vi "ReadStrains_v200128_A.vi"() -> ()   [LabVIEW 2017]
doc: "I. Description:\nThis example demonstrates how to make continuous, hardware-timed temperature measurement using a thermocouple.\n\nII. Instructions for Running:\n1. Specify the Physical Channel where you have connected the thermocouple.\n2. Enter the Minimum and Maximum temperature values in degrees C you expect to measure. A smaller range will allow a more accurate measurement.\n3. Enter the scan rate at which you want to run the acquisition.\n4. Specify the type of thermocouple you are using.\n5. Thermocouple measurements require cold-junction compensation (CJC) to correctly scale them. Specify the source of your cold-junction compensation.\n6. If your CJC source is \"Internal\", skip the rest of the steps.\n7. If your CJC source is \"Constant Value\", specify the value (usually room temperature) in degrees C.\n8. If your CJC source is \"Channel\", specify the CJC Channel name. \n9. Specify the appropriate Auto Zero Mode. See your device's hardware manual to find out if your device supports this attribute.\n\nIII. Block Diagram Steps:\n1. Create a Thermocouple (TC) temperature measurement channel.\n2. Get all the channels in the task.\n3. Convert channel(s) array to a comma-delimited channel string.\n4. This attribute is set to compensate for input offset errors. May not be supported by all devices*.\n5. Call the Timing VI to specify the hardware timing parameters. Use device's internal clock, continuous mode acquisition and the sample rate specified by the user.\n6. Call the Start VI to program and start the acquisition.\n7. Read N samples and plot it. By default, the Read VI reads all available samples, but you can specify how many samples to read at a time and the timeout value. Continue reading data until the stop button is pressed or an error occurs. \n8. Call the Clear Task VI to clear the Task.\n9. Use the popup dialog box to display an error if any.\n\n* If your device does not support Auto Zero Mode bypass Step 2, 3, and 4.\n\nIV. I/O Connections Overview:\nConnect your thermocouple to the terminals corresponding to the Physical Channel I/O Control value."
uses:
  <vilib>/Utility/error.llb/DialogType.ctl
  <vilib>/DAQmx/read.llb/DAQmx Read (Analog 1D Wfm NChan NSamp).vi
  <vilib>/Analysis/baseanly.llb/Mean (DBL).vi
  <vilib>/Waveform/WDTOps.llb/WDT Index Channel DBL.vi
  <vilib>/DAQmx/create/channels.llb/DAQmx Create Channel (AI-Voltage-Basic).vi
  <vilib>/DAQmx/configure/timing.llb/DAQmx Timing (Sample Clock).vi
  <vilib>/DAQmx/miscellaneous.llb/DAQmx Fill In Error Info.vi
  <vilib>/Analysis/NI_AALBase.lvlib
  <vilib>/ptbypt/NI_PtbyPt.lvlib
  <vilib>/Utility/miscctls.llb/LVRowAndColumnTypeDef.ctl
panel:
  in  "Data Tag":dbl=99.0 format="%.2p"
  out "Load Cell Min Peak":dbl format="%0.2f"
  out "Load Cell Max Peak":dbl format="%0.2f"
  in  "Stop":bool
  in  "Color Box":u32(colorbox)=16448250
  out "Results":i32[](listbox)
  in  "num_chans":i32=4
  in  "Search Strings":string[](array[string])=["Verbose Name", "Units", "Sensitivity", "Offset"]
  out "TRQ_2SPD_OT (N·m)":dbl=-0.01305389404296875 format="%0.3f"
  out "Power_OT (W)":dbl=-4.779110606064606 format="%.2f"
  out "rpm_out/rpm_in":dbl=-8.382425226893735e-05 format="%.3g"
  out "AI Consumer Iterations":i32=46
  in  "path":path=path "D:/LabView Data"
  out "P2 - P1":dbl=2.2560862731933593 format="%.3f"
  out "Recorded Blocks":dbl=46.0
  in  "Force Record":bool caption="Force Record Enable"
  out "data 2":waveform(dbl)[](array[waveform])=[{"t0"=timestamp(3650018127.9917235 s since 1904-01-01), "dt"=0.1, "Y"=[0.021594634133905076, 0.022275858634939055], "attributes"=variant("NI_ChannelName"=variant(string "Dev1/ai0"), "NI_UnitDescription"=variant(string "Volts"))}, {"t0"=timestamp(3650018127.9917235 s since 1904-01-01), "dt"=0.1, "Y"=[2.0002340930725198, 1.9998772609501023], "attributes"=variant("NI_ChannelName"=variant(string "Dev1/ai0"), "NI_UnitDescription"=variant(string "Volts"))}, {"t0"=timestamp(3650018127.9917235 s since 1904-01-01), "dt"=0.1, "Y"=[1.9878001157523826, 1.9871643057998443], "attributes"=variant("NI_ChannelName"=variant(string "Dev1/ai0"), "NI_UnitDescription"=variant(string "Volts"))}, {"t0"=timestamp(3650018127.9917235 s since 1904-01-01), "dt"=0.1, "Y"=[0.006912624203864532, 0.006889916720453561], "attributes"=variant("NI_ChannelName"=variant(string "Dev1/ai0"), "NI_UnitDescription"=variant(string "Volts"))}, {"t0"=timestamp(3650018127.9917235 s since 1904-01-01), "dt"=0.1, "Y"=[0.0, 0.0], "attributes"=variant("NI_ChannelName"=variant(string "Dev1/ai0"), "NI_UnitDescription"=variant(string "Volts"))}]
  out "Power_IN (W)":dbl=0.0005711775684961294 format="%.2g"
  out "TRQ_2SPD_DRVLN_OT (N·m)":dbl=-0.018612060546874976 format="%0.3f"
  out "Waveform Chart":waveform(dbl)[](graph)=[{"t0"=timestamp(3663084502.027375 s since 1904-01-01), "dt"=0.1, "Y"=[-0.17066702696318498, -0.13693019437081472], "attributes"=variant("NI_ChannelName"=variant(string "HS_2210_STRAIN_A_POUNDS"), "NI_UnitDescription"=variant(string "lbf"))}, {"t0"=timestamp(3663084502.027375 s since 1904-01-01), "dt"=0.1, "Y"=[-50.01120067249004, -50.01071408355846], "attributes"=variant("NI_ChannelName"=variant(string "T1_OIL_OT"), "NI_UnitDescription"=variant(string "°C"))}, {"t0"=timestamp(3663084502.027375 s since 1904-01-01), "dt"=0.1, "Y"=[-0.013838771793185324, -0.013803088604682188], "attributes"=variant("NI_ChannelName"=variant(string "HS_2210_STRAIN_B_VOLTS"), "NI_UnitDescription"=variant(string "V"))}, {"t0"=timestamp(3663084502.027375 s since 1904-01-01), "dt"=0.1, "Y"=[10.033860995992347, 10.033912900500356], "attributes"=variant("NI_ChannelName"=variant(string "HS_2210_EXC_B_VOLTS"), "NI_UnitDescription"=variant(string "V"))}, {"t0"=timestamp(3663084502.027375 s since 1904-01-01), "dt"=0.1, "Y"=[1.48, 1.48], "attributes"=variant("NI_ChannelName"=variant(string "RPM_RATIO"), "NI_UnitDescription"=variant(string "ratio"))}, {"t0"=timestamp(3663084502.027375 s since 1904-01-01), "dt"=0.1, "Y"=[99.0, 99.0], "attributes"=variant("NI_ChannelName"=variant(string "DataTag"), "NI_UnitDescription"=variant(string "none"))}, {"t0"=timestamp(3663084502.027375 s since 1904-01-01), "dt"=0.1, "Y"=[0.0, 0.0], "attributes"=variant("NI_ChannelName"=variant(string "LV_CMD_2SPD_OIL_SLND"), "NI_UnitDescription"=variant(string "boolean"))}]
  in  "Run Letter":string="a"
  out "Recording":bool
  in  "Num_Blocks":dbl=100.0
  in  "Maximum Value":dbl=10.0 format="%0.2f"
  in  "Minimum Value":dbl=-10.0 format="%0.2f"
  in  "Physical Channel":tag="Dev1/ai0:3" caption="PCI-6143_1 Channels"
  in  "Rate":dbl=1000.0 format="%0.2f"
  # "rev 150415_A  added \"Record Run X\" sub VI.\nrev 150423_A added power, efficiency, and manual inputs for speed .\nrev 150423_B added speed measurement via PCI-6602 card.\nrev 161117_A is set up for the alternator test reading shaft RPM from Dynapar encoder and torque from the Omega TQ513-1K paired with the Omega DP41-S.\nrev 170504_A migrated DAQ h/w from the SCXI chassis (now being used for TC2 porcupine testing) to PCI-6143.\nrev 170510_A takes data at 1000Hz, then averages groups of 100 samples for a logging rate of 10Hz per channel.  Added function that resets \"Data Tag\"\nto 99 after \"Num_Blocks\" has been recorded.\nrev 170810_A adds flowmeter for 2-speed supercharger drive bench test.  CJP\nrev 170821_A logs tags to same file for a given run letter.  Uses \"Record Continuous Tags...\" sub VI.\nrev 171129_A is for the Orthrus 2-speed drive.  Added new encoder period measurement for the 127 tooth geat \"RPM_2SPD_OT\". CJP\nrev 171130_A adds Digital Output (DO) for 2SPD drive control.  Will log this with the rest of the data.  Also corrected the number of teeth on the 2SPD Output side from 127 to 107!\nrev 171201_A restructuring for  \"real-time\" response to speed changes by moving the disklog to a separate loop (queue).\nrev 171201_B moves counters into main AI loop and adds a start trigger so DAQ won't start until rig is spinning.  Added F-V where old \"F1\" channel was for \"RPM_2SPD_OT\".   CJP\nrev 171201_C uses a CI-Frequency task for RPM instead of period.  Testing this for better transient response.  This appears to be even slower than the period measurement.\nrev 171201_D is built from rev 171201_A, but adding in the F-V channel.  This version queues both the AI channel and CI channels to a single Consumer.  Also adding a 30s switch to automate switching of the 2SPD solenoid.\nrev 171221_A was the first attempt at this and for some reason, while running that VI, the computer froze, unable to do ctrl+alt+del reboot.  After rebooting, the VI was no longer openable in LabView 2014 or LabView 2016.  Will try the same process over with v171226_A.\nrev 171226_A adds one more PCI_6143 card for 8 additional analog inputs.\nrev 171226_B created a backup with 171226_A.\nrev 180314_A added thermocouple for Sumanth.  This is for testing the 2-Speed Drive.\nrev Read \"ThermVolt_TestSpeed_180406_A.vi\" is for verifying the one remaining Micro-Epsilon speed sensor on the 2Spd Drive.\nrev \"Read Thermocouples and Voltages v180406_A.vi\" reintroduces the two counter/timer channels on the PCI-6602 card for the driveline encoder and \nMicro-Epsilon 2Spd Output.\nrev 180919_A built off of rev 180426_A for 2-Speed Drive testing.  CJP\nv181002_A adding new T22 at 2SPD input pulley AND keeping original T22 at output end of drivline.  CJP\nv181004_A corrected front panel displays for Power_IN and Power_OT.  CJP\nv181025_A adding ReadChnCfg.VI to read channel names, units, scaling, and offset from Labview Channel Map\nv190401_A restructuring \"Read Thermocouples and Voltages...\" to use only channels from NI-6229 out of test cell 2.  CJP\nv190516_A adds frequency measurement for driveline speed since F-V measurements not working.  CJP"
  # "For instructions, select Help>>Show Context Help"
  # "Now using 360 PPR encoder for input speed 171227.\nChanged to Input Gear Speed 180118.  CJP  127 Hz = 1 RPS, 127 Hz = 60 RPM\n5 kHz = 1 V => 5000/127 = 39.37 RPS = 2362.205 RPM\nv180314_A 5kHz = 1V = 5000/360 = 13.888 RPS = 833.33 RPM.\nBack to 360PPR encoder with pulley ratio of 1.48."
  # "HBM T21WN"
  # "Interface T22"
  # "Timing Parameters"
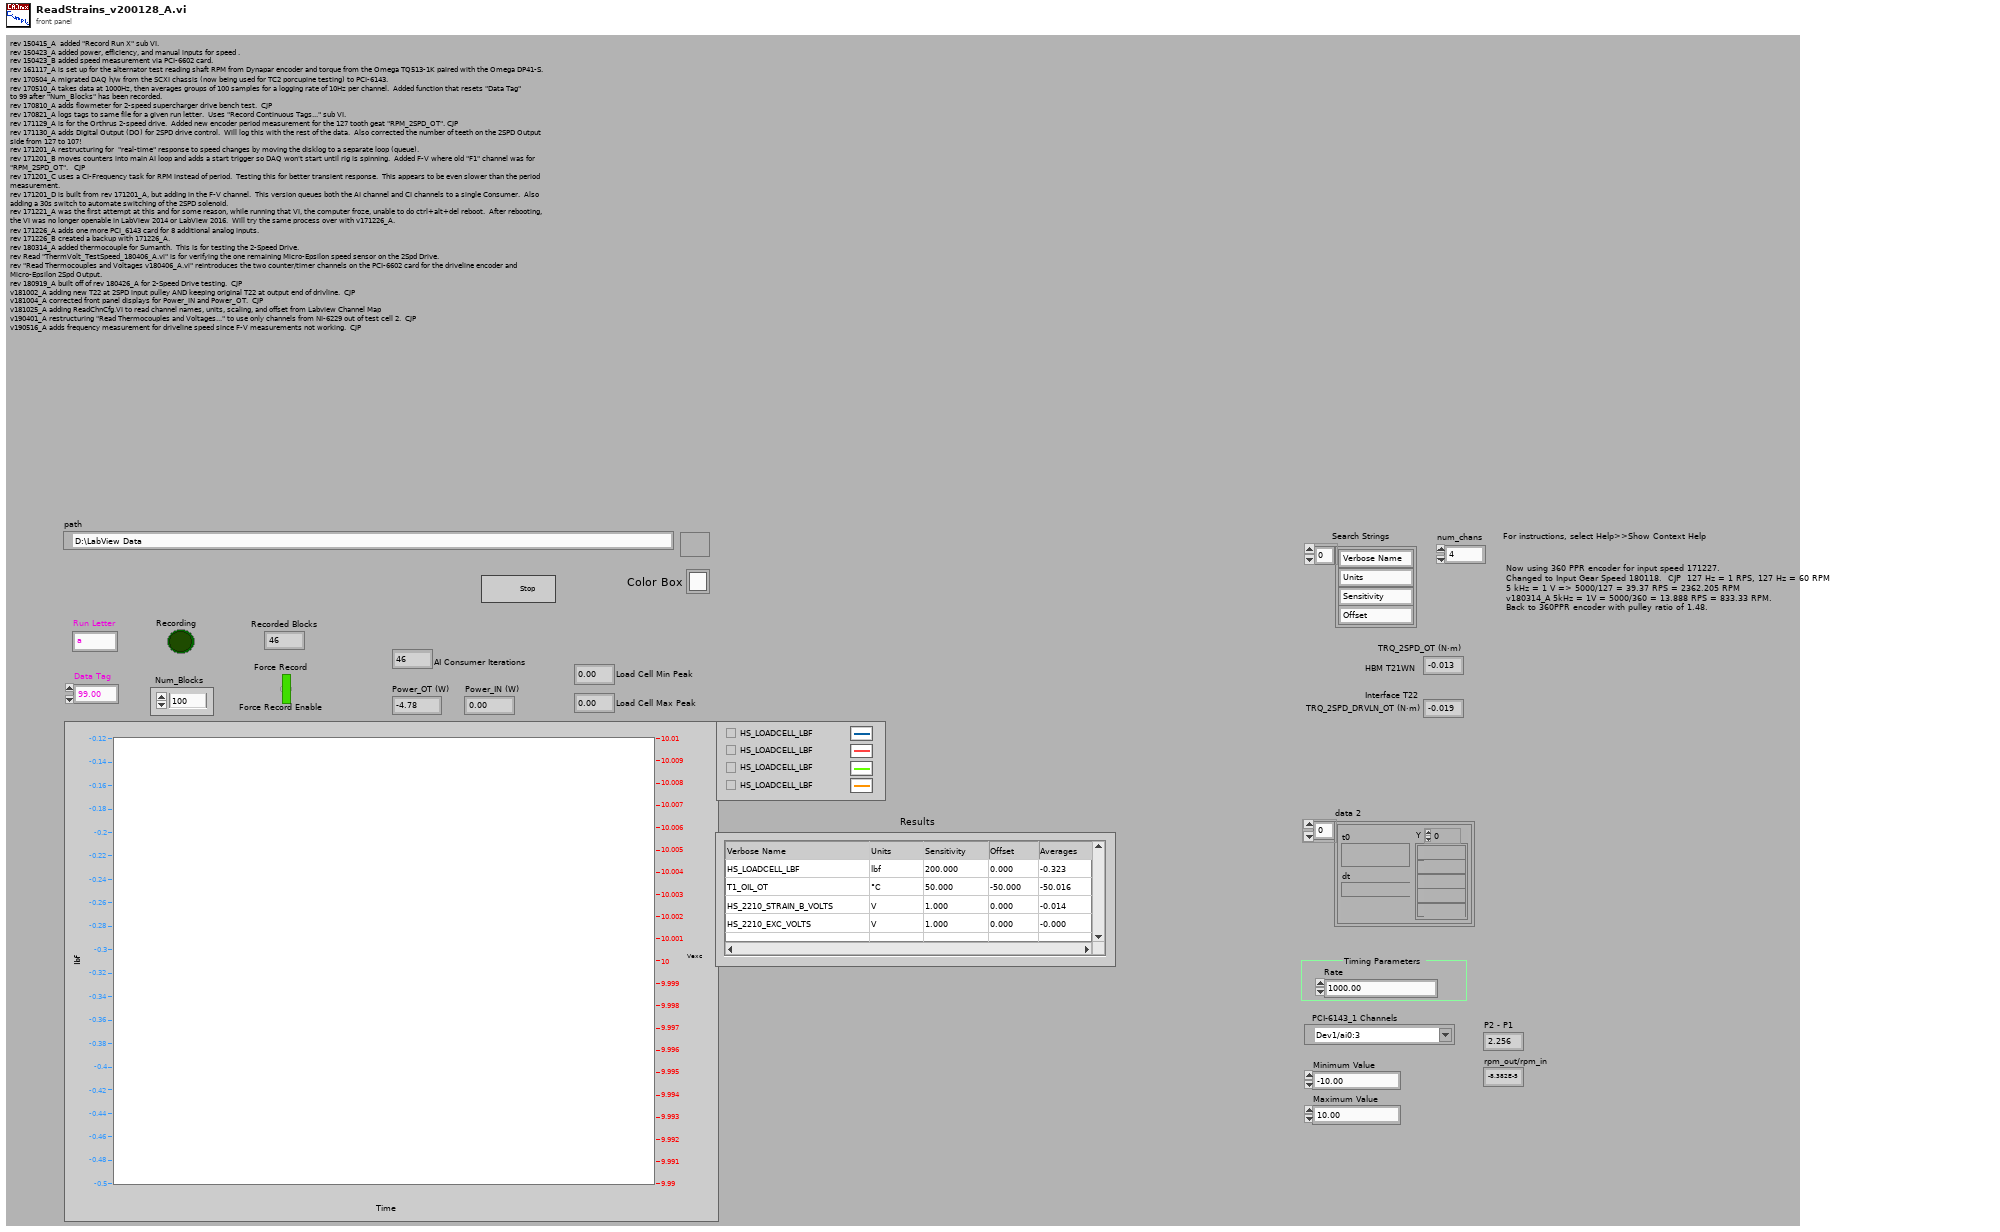
[diagram p1: front panel]
types:
  T1 = typedef "DialogType.ctl" = u16
  T2 = typedef "LVRowAndColumnTypeDef.ctl" = cluster{"Row":i32, "Column":i32}
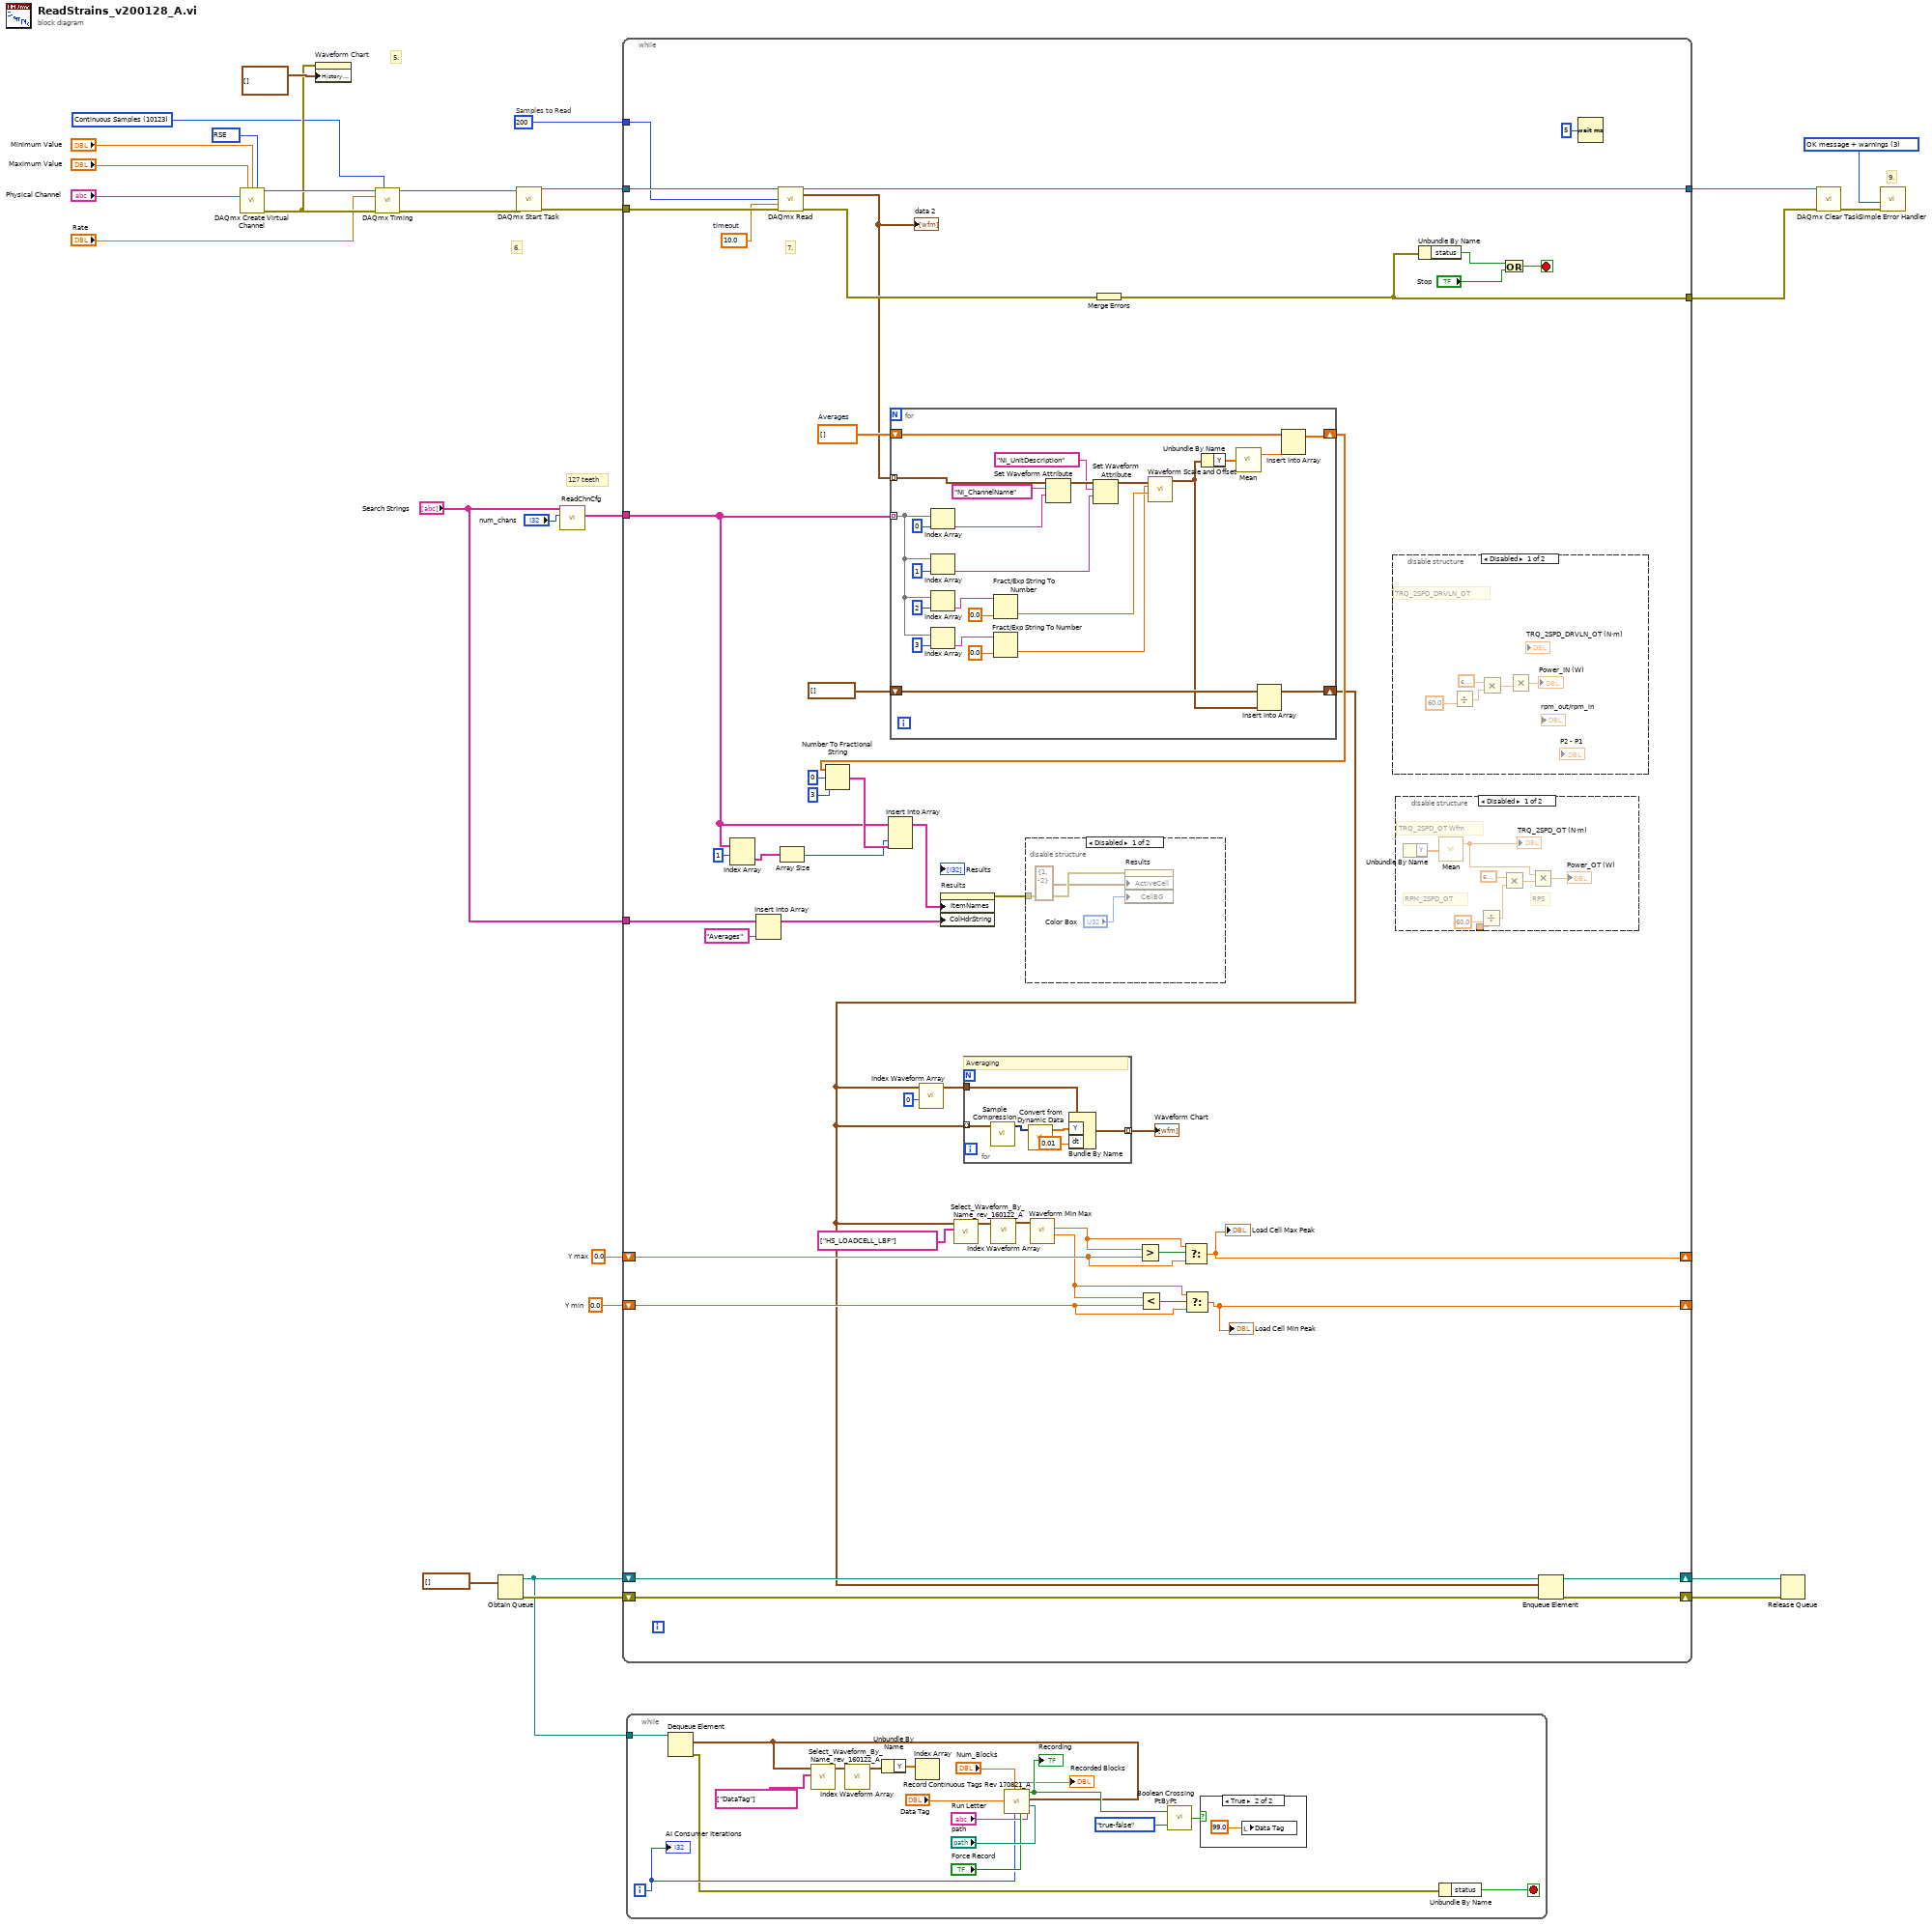
[diagram p0: block diagram]
diagram:
  w1 = 0.0  # Y min
  w2 = 0.0  # Y max
  w3 = 10083 items=["Default"=-1, "RSE"=10083, "NRSE"=10078, "Differential"=10106, "Pseudodifferential"=12529] ("input terminal configuration")
  w23 = T1 3 items=["no dialog", "OK message", "continue or stop message", "OK message + warnings", "continue/stop + warnings"] ("type of dialog (OK msg:1)")
  w9 = 10123 items=["Finite Samples"=10178, "Continuous Samples"=10123] ("sample mode")
  # "127 teeth"
  # "Samples to Read"
  # "9."
  # "5."
  # "6."
  n1 = call-poly <vilib>:"DAQmx Create Virtual Channel.vi"("maximum value"="Maximum Value", "minimum value"="Minimum Value", "input terminal configuration"=w3, "physical channels"="Physical Channel") -> ("task out"=w21:refnum<k21>, "error out"=w19:errorcluster)  [unwired: 10 in]
  n2 = property on="Waveform Chart" class="WFChart (strict)"(error in=w19, "History Data"=waveform(dbl)[][] []) -> ()  [unwired: 1 in, 2 out]
  n3 = call-poly <vilib>:"DAQmx Timing.vi"("task/channels in"=w21, "sample mode"=w9, "rate"="Rate", "error in"=w19) -> ("task out"=w24:refnum<k21>, "error out"=w4:errorcluster)  [unwired: 10 in]
  n4 = Obtain Queue(element data type=waveform(dbl)[] [] ("appended array")) -> (queue out=w13:refnum<queue>, error out=w16:errorcluster)  [unwired: 4 in, 1 out]
  n5 = call <vilib>:"DAQmx Start Task.vi"("task/channels in"=w24, "error in"=w4) -> ("task out"=w26:refnum<k21>, "error out"=w27:errorcluster)  [unwired: 12 in]
  n6 = call "ReadChnCfg.vi"("num_chans"="num_chans", "Search Strings"="Search Strings") -> ("Table Minus Headers"=w7:string[][])  [unwired: 8 in, 1 out]
  n7 = while {
    tunnel: w26 -> [w74]
    tunnel: w27 -> [w73]
    tunnel: [w72] -> w25
    tunnel: 200 ("number of samples per channel") -> [w45]
    shift-right: [w64] -> w15
    shift-left: w13 -> [w66]
    shift-right: [w63] -> w14
    shift-left: w16 -> [w65]
    tunnel: [w47] -> w5
    tunnel: w7 -> [w50]
    tunnel: "Search Strings" -> [w60]
    shift-right: [w34] -> _
    shift-left: w2 -> [w35]
    shift-right: [w31] -> _
    shift-left: w1 -> [w30]
    stop <- w69 stop-if-true
    w62 = dbl[] []  # Averages
    w70 = 10.0  # timeout
    # "7."
    n8 = Index Array(array=w50, index (row)=1) -> (element=w54:string[])  [unwired: 1 in]
    n9 = Insert Into Array(array=w60, new element="Averages" ("new element/subarray")) -> (w51:string[])  [unwired: 1 in]
    n10 = call-poly <vilib>:"DAQmx Read.vi"("task/channels in"=w74, "number of samples per channel"=w45, "timeout"=w70, "error in"=w73) -> ("task out"=w72:refnum<k21>, "data"=w42:waveform(dbl)[], "error out"=w48:errorcluster)  [unwired: 9 in]
    "data 2" <- w42
    n11 = Array Size(array=w54) -> (size(s)=w53:i32)
    n12 = for {
      tunnel: w42 -> [w108] mode=indexing
      shift-right: [w107] -> w43
      shift-left: w62 -> [w106]
      tunnel: w50 -> [w95] mode=indexing
      shift-right: [w102] -> w29
      shift-left: waveform(dbl)[] [] -> [w104]
      n13 = Index Array(array=w95, index=0) -> (element=w99:string)
      n14 = Index Array(array=w95, index=1) -> (element=w98:string)
      n15 = Index Array(array=w95, index=2) -> (element=w94:string)
      n16 = Index Array(array=w95, index=3) -> (element=w90:string)
      n17 = Fract/Exp String To Number(string=w94, default (0 dbl)=0.0) -> (number=w92:dbl)  [unwired: 2 in, 1 out]
      n18 = Fract/Exp String To Number(string=w90, default (0 dbl)=0.0) -> (number=w89:dbl)  [unwired: 2 in, 1 out]
      n19 = Set Waveform Attribute(5:w99, 6:"NI_ChannelName" ("name"), 7:w108) -> (3:w112:waveform(dbl))  [unwired: 1 in, 2 out]
      n20 = Set Waveform Attribute(5:w98, 6:"NI_UnitDescription" ("name"), 7:w112) -> (3:w110:waveform(dbl))  [unwired: 1 in, 2 out]
      n21 = call <vilib>:"Waveform Scale and Offset.vi"("scale"=w92, "offset"=w89, "waveform in"=w110) -> ("waveform out"=w103:waveform(dbl))  [unwired: 7 in, 1 out]
      n22 = Unbundle By Name(w103) -> ("Y"=w109:dbl[])
      n23 = call-poly <vilib>:"Mean.vi"("X"=w109) -> ("mean"=w105:dbl)  [unwired: 1 out]
      n24 = Insert Into Array(array=w104, new element=w103) -> (w102:waveform(dbl)[])  [unwired: 1 in]
      n25 = Insert Into Array(array=w106, new element=w105) -> (w107:dbl[])  [unwired: 1 in]
    }
    n26 = Number To Fractional String(number=w43, width (-)=i16 0, precision (6)=i16 3) -> (F-format string=w56:string[])  [unwired: 1 in]
    n27 = Insert Into Array(array=w50, index (col)=w53, new element=w56) -> (w52:string[][])  [unwired: 1 in]
    n28 = call-poly <vilib>:"Index Waveform Array.vi"("index"=0, "waveform array"=w29) -> ("waveform"=w44:waveform(dbl))  [unwired: 8 in, 1 out]
    n29 = property on="Results" class="MCListbox (strict)"("ItemNames"=w52, "ColHdrString"=w51) -> (error out=w49:errorcluster)  [unwired: 2 in, 1 out]
    n30 = call "Select_Waveform_By_Name_rev_160122_A.vi"("Array"=string[] ["HS_LOADCELL_LBF"], "Waveform Array"=w29) -> ("Array 2"=w39:waveform(dbl)[])  [unwired: 9 in]
    n31 = for {
      tunnel: w29 -> [w80] mode=indexing
      tunnel: [w79] -> w41 mode=indexing
      tunnel: w44 -> [w78]
      # "Averaging"
      n32 = call "Sample Compression"("Signals"=w80) -> ("Mean"=w81:dynamicdata)  [unwired: 8 in, 2 out]
      n33 = call "Convert from Dynamic Data"("Dynamic Data Type"=w81) -> ("Array"=w83:dbl[])  [unwired: 3 in]
      n34 = Bundle By Name(cluster=w78, "Y"=w83, "dt"=0.01) -> (w79:waveform(dbl))
    }
    "Waveform Chart" <- w41
    n35 = call-poly <vilib>:"Index Waveform Array.vi"("waveform array"=w39) -> ("waveform"=w38:waveform(dbl))  [unwired: 9 in, 1 out]
    n36 = disable-structure shown="Disabled" {
      disable-tunnel: w49 -> [w77 _]
      frame Disabled {
        n37 = property on="Results" class="MCListbox (strict)"(error in=w77, "ActiveCell"=T2 {"Row"=1, "Column"=-2} ("Active Cell:Active Cell"), "CellBG"="Color Box") -> ()  [unwired: 1 in, 2 out]
      }
      frame Enabled {
      }
    }
    n38 = call <vilib>:"Waveform Min Max.vi"("waveform in"=w38) -> ("Y min"=w32:dbl, "Y max"=w36:dbl)  [unwired: 5 in, 4 out]
    n39 = Merge Errors(w48) -> (w47:errorcluster)
    n40 = Greater?(x=w36, y=w35) -> (0:w37:bool)
    n41 = Less?(x=w32, y=w30) -> (x < y?=w33:bool)
    n42 = Select(t=w36, s=w37, f=w35) -> (s? t:f=w34:dbl)
    "Load Cell Max Peak" <- w34
    n43 = Select(t=w32, s=w33, f=w30) -> (s? t:f=w31:dbl)
    "Load Cell Min Peak" <- w31
    n44 = disable-structure shown="Disabled" {
      frame Disabled {
        # "TRQ_2SPD_DRVLN_OT"
        n45 = Divide(y=60.0) -> (x/y=w84:dbl)  [unwired: 1 in]
        n46 = Multiply(x=6.283185307179586, y=w84) -> (x*y=w87:dbl)
        n47 = Multiply(y=w87) -> (x*y=→"Power_IN (W)":dbl)  [unwired: 1 in]
      }
      frame Enabled {
      }
    }
    n48 = disable-structure shown="Disabled" {
      disable-tunnel: _ -> [w114 _]
      frame Disabled {
        # "RPM_2SPD_OT"
        # "TRQ_2SPD_OT Wfm"
        # "RPS"
        n49 = Unbundle By Name() -> ("Y"=w118:dbl[])  [unwired: 1 in]
        n50 = call-poly <vilib>:"Mean.vi"("X"=w118) -> ("mean"=w117:dbl)  [unwired: 1 out]
        "TRQ_2SPD_OT (N·m)" <- w117
        n51 = Divide(x=w114, y=60.0) -> (x/y=w115:dbl)
        n52 = Multiply(x=6.283185307179586, y=w115) -> (x*y=w120:dbl)
        n53 = Multiply(x=w117, y=w120) -> (x*y=→"Power_OT (W)":dbl)
      }
      frame Enabled {
      }
    }
    n54 = Unbundle By Name(w47) -> ("status"=w71:bool)
    n55 = Or(x=w71, y="Stop") -> (x .or. y?=w69:bool)
    n56 = Enqueue Element(queue=w66, element=w29, error in (no error)=w65) -> (queue out=w64:refnum<queue>, error out=w63:errorcluster)  [unwired: 1 in, 1 out]
    n57 = Wait (ms)(milliseconds to wait=u32 5) -> ()  [unwired: 1 out]
  }
  n58 = while {
    tunnel: w13 -> [w131]
    i -> [w130]
    stop <- w123 stop-if-true
    n59 = Dequeue Element(queue=w131) -> (element=w125:waveform(dbl)[], error out=w124:errorcluster)  [unwired: 2 in, 2 out]
    n60 = call "Select_Waveform_By_Name_rev_160122_A.vi"("Array"=string[] ["DataTag"], "Waveform Array"=w125) -> ("Array 2"=w128:waveform(dbl)[])  [unwired: 9 in]
    n61 = call-poly <vilib>:"Index Waveform Array.vi"("waveform array"=w128) -> ("waveform"=w127:waveform(dbl))  [unwired: 9 in, 1 out]
    n62 = Unbundle By Name(w127) -> ("Y"=w126:dbl[])
    n63 = Index Array(array=w126) -> ()  [unwired: 1 in, 1 out]
    n64 = call "Record Continuous Tags Rev 170821_A.vi"("Run Letter"="Run Letter", "path"="path", "Waveform Array In"=w125, "Force Record"="Force Record", "Main Count"=w130, "Num_Blocks"="Num_Blocks", "Data Tag"="Data Tag") -> ("Record Cmd"=w137:bool, "Recorded Blocks"=→"Recorded Blocks":dbl)  [unwired: 2 in, 1 out]
    "Recording" <- w137
    n65 = call <vilib>:"Boolean Crossing PtByPt.vi"("direction"=enum16{"either", "false-true", "true-false"}."true-false", "input"=w137) -> ("crossing"=w138:bool)  [unwired: 1 in]
    n66 = case shown="True" w138 {
      frame False {
      }
      frame True {
        n67 = local write "Data Tag"(99.0 ("y")) -> ()
      }
    }
    n68 = Unbundle By Name(w124) -> ("status"=w123:bool)
    "AI Consumer Iterations" <- w130
  }
  n69 = Release Queue(queue=w15, error in (no error)=w14) -> ()  [unwired: 1 in, 3 out]
  n70 = call <vilib>:"DAQmx Clear Task.vi"("task in"=w25, "error in"=w5) -> ("error out"=w28:errorcluster)  [unwired: 13 in]
  n71 = call <vilib>:"Simple Error Handler.vi"("type of dialog (OK msg:1)"=w23, "error in (no error)"=w28) -> ()  [unwired: 3 in, 5 out]
